vi "ADIS16448 Process Example.vi"(8 "error in (no error)":errorcluster, 11 "output":T1) -> (0 "error out":errorcluster)   [LabVIEW 2025]
uses:
  <vilib>/Rock Robotics/WPI/ThirdParty/ADI/ADIS16448/Typedef/ADIS16448 Data.ctl
  <vilib>/ptbypt/NI_PtbyPt.lvlib
panel:
  out "Average Time Delta":dbl
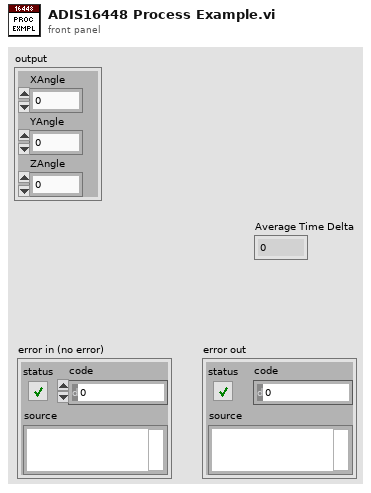
[diagram p1: front panel]
types:
  T1 = typedef "ADIS16448 Data.ctl" = cluster{"XAngle":dbl, "YAngle":dbl, "ZAngle":dbl}
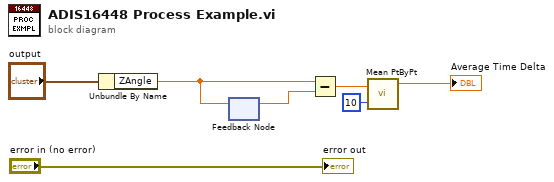
[diagram p0: block diagram]
diagram:
  n1 = Unbundle By Name("output") -> ("ZAngle"=w6:dbl)
  n2 = feedback-in #1(w6) -> ()
  n3 = feedback #1() -> (w5:dbl)  [unwired: 1 in]
  n4 = Subtract(x=w6, y=w5) -> (x-y=w4:dbl)
  n5 = call <vilib>:"Mean PtByPt.vi"("x"=w4, "sample length"=10) -> ("mean"=→"Average Time Delta":dbl)  [unwired: 2 in, 1 out]
  "error out" <- "error in (no error)"
